vi "PantherLAB_Log - Create RT Tester.vi"(11 "Module Info":T1) -> (0 "error out":errorcluster)   [LabVIEW 2016]
doc: "_____\nCreated using DQMH Framework: Event Scripter 7.1.0.1450."
uses:
  <vilib>/Delacor/Delacor QMH/Libraries/_Scripting Support/Module Info--cluster.ctl
  <vilib>/Delacor/Delacor QMH/Libraries/_Scripting Support/Module Type--enum.ctl
  PantherLAB Scripting Hooks/PantherLAB_Scripting.lvlib
  <vilib>/Delacor/Delacor QMH/Libraries/_Scripting Support/dqmh_lib_DQMH Scripting Support.lvlib
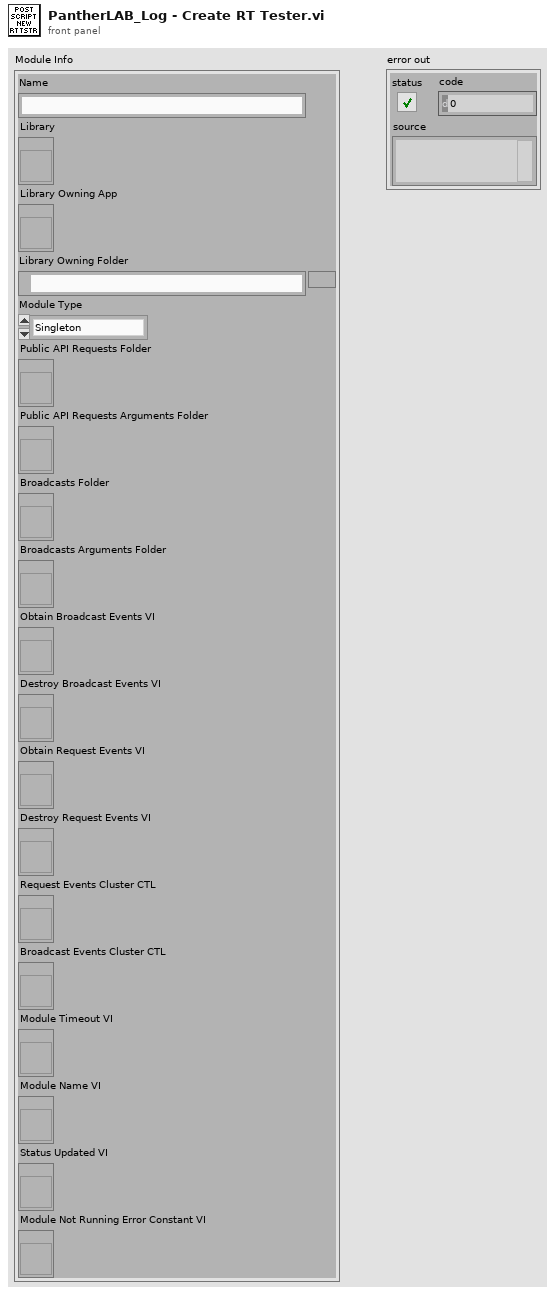
[diagram p1: front panel]
types:
  T1 = typedef "dqmh_lib_DQMH Scripting Support.lvlib/Module Info--cluster.ctl" = cluster{"Name":string, "Library":refnum<vi>, "Library Owning App":refnum<vi>, "Library Owning Folder":path, "Module Type":T2, "Public API Requests Folder":refnum<vi>, "Public API Requests Arguments Folder":refnum<vi>, "Broadcasts Folder":refnum<vi>, "Broadcasts Arguments Folder":refnum<vi>, "Obtain Broadcast Events VI":refnum<vi>, "Destroy Broadcast Events VI":refnum<vi>, "Obtain Request Events VI":refnum<vi>, "Destroy Request Events VI":refnum<vi>, "Request Events Cluster CTL":refnum<vi>, "Broadcast Events Cluster CTL":refnum<vi>, "Module Timeout VI":refnum<vi>, "Module Name VI":refnum<vi>, "Status Updated VI":refnum<vi>, "Module Not Running Error Constant VI":refnum<vi>}
  T2 = typedef "dqmh_lib_DQMH Scripting Support.lvlib/Module Type--enum.ctl" = enum16{"Singleton", "Cloneable"}
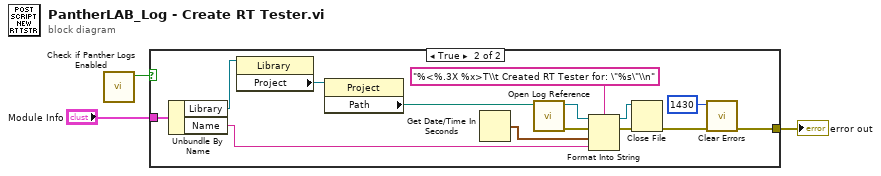
[diagram p0: block diagram]
diagram:
  n1 = call "Check if Panther Logs Enabled.vi"() -> ("PantherLogs Enabled?"=w2:bool)  [unwired: 11 in]
  n2 = case shown="True" w2 {
    tunnel: [_ w5] -> w3
    tunnel: "Module Info" -> [_ w14]
    frame False {
    }
    frame True {
      n3 = Unbundle By Name(w14) -> ("Library"=w13:refnum<vi>, "Name"=w9:string)
      n4 = property class="Library"(reference=w13) -> ("Project"=w12:refnum<vi>)  [unwired: 1 in, 2 out]
      n5 = property class="Project"(reference=w12) -> ("Path"=w7:path)  [unwired: 1 in, 2 out]
      n6 = Get Date/Time In Seconds() -> (seconds since 1Jan1904=w8:timestamp)
      n7 = call "Open Log Reference.vi"("Project Path"=w7) -> ("error out"=w17:errorcluster, "File Reference"=w11:refnum<file>)  [unwired: 9 in]
      n8 = Format Into String(format string="%<%.3X %x>T\\t Created RT Tester for: \"%s\"\\n", initial string=w11, error in=w17, w8, w9) -> (resulting string=w10:refnum<file>, error out=w16:errorcluster)
      n9 = Close File(refnum=w10, error in=w16) -> (error out=w15:errorcluster)  [unwired: 1 out]
      n10 = call <vilib>:"Clear Errors.vi"("error in (no error)"=w15, "specific error code to clear (0: all)"=1430) -> ("error out"=w5:errorcluster)  [unwired: 4 in, 1 out]
    }
  }
  "error out" <- w3
